vi "Simple Test.vi"() -> ()   [LabVIEW 2019, in "instrument.PPMS.lvclass"]
uses:
  instrument.PPMS.lvclass
  PPMS/Select PPMS--Enum.ctl
  PPMS/PPMS.lvlib
panel:
  out "x-y":dbl
  out "Temperature (K)":dbl
  in  "stop":bool
  in  "Select PPMS":T1=enum."Simulate PPMS"
  out "Paths":string
  out "getAll":variant
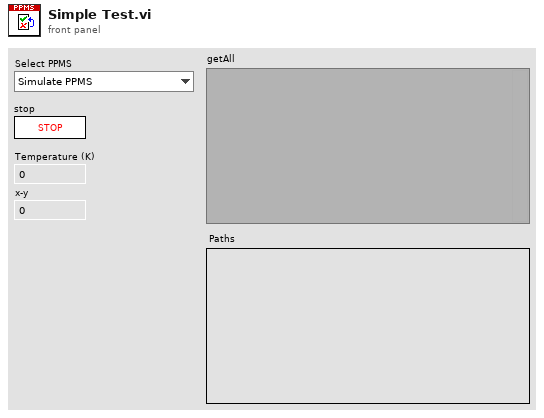
[diagram p1: front panel]
types:
  T1 = typedef "PPMS.lvlib/Select PPMS--Enum.ctl" = enum16{"PPMS1", "PPMS2", "PPMS3", "OptiCool", "Simulate PPMS", "Simulate OptiCool"}
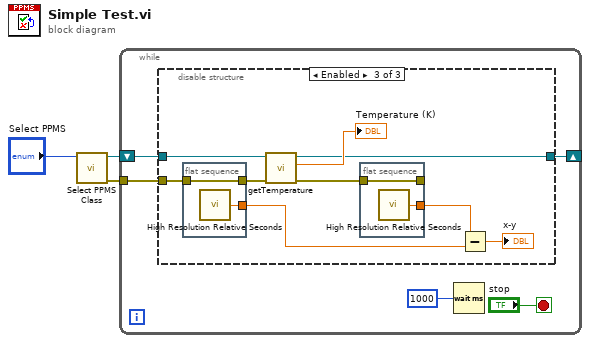
[diagram p0: block diagram]
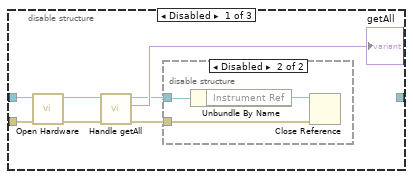
[diagram p2: hidden frame]
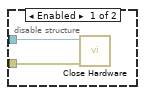
[diagram p3: hidden frame]
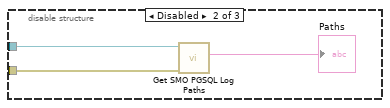
[diagram p4: hidden frame]
diagram:
  n1 = call "Select PPMS Class.vi"("Select PPMS"="Select PPMS") -> ("error out"=w2:errorcluster, "instrument.PPMS out"=w3:refnum<class "instrument.PPMS.lvclass">)  [unwired: 9 in]
  n2 = while {
    tunnel: w2 -> [w7]
    shift-right: [w5] -> _
    shift-left: w3 -> [w8]
    stop <- "stop" stop-if-true
    n3 = disable-structure shown="Enabled" {
      disable-tunnel: w8 -> [w15 w23 w32]
      disable-tunnel: w7 -> [w14 w22 w29]
      disable-tunnel: [_ _ w28] -> w5
      frame Disabled {
        n4 = call-dynamic "Open Hardware.vi"("error in (no error)"=w14, "instrument.PPMS"=w15) -> ("error out"=w12:errorcluster, "instrument.PPMS out"=w13:refnum<class "instrument.PPMS.lvclass">)  [unwired: 8 in]
        n5 = call-dynamic "Handle getAll.vi"("error in (no error)"=w12, "instrument.PPMS in"=w13) -> ("error out"=w11:errorcluster, "getAll"=→"getAll":variant, "instrument.PPMS out"=w9:refnum<class "instrument.PPMS.lvclass">)  [unwired: 7 in]
        n6 = disable-structure shown="Disabled" {
          disable-tunnel: w11 -> [w17 w20]
          disable-tunnel: w9 -> [w16 w19]
          frame Enabled {
            n7 = call-dynamic "Close Hardware.vi"("error in (no error)"=w17, "instrument.PPMS"=w16) -> ()  [unwired: 8 in, 2 out]
          }
          frame Disabled {
            n8 = Unbundle By Name(w19) -> ("Instrument Ref"=w18:refnum<k24>)
            n9 = Close Reference(reference=w18, error in (no error)=w20) -> ()  [unwired: 1 out]
          }
        }
      }
      frame Disabled {
        n10 = call-dynamic "Get SMO PGSQL Log Paths.vi"("error in (no error)"=w22, "Instrument in"=w23) -> ("Paths"=→"Paths":string)  [unwired: 7 in, 2 out]
      }
      frame Enabled {
        n11 = flat-sequence {
          tunnel: [w36] -> w30
          tunnel: w29 -> [w36]
          tunnel: [w35] -> w24
          frame #0 {
            n12 = call <vilib>:"High Resolution Relative Seconds.vi"() -> ("relative seconds"=w35:dbl)
          }
        }
        n13 = call-dynamic "getTemperature.vi"("error in (no error)"=w30, "instrument.PPMS"=w32) -> ("error out"=w27:errorcluster, "Temperature (K)"=→"Temperature (K)":dbl, "instrument.PPMS out"=w28:refnum<class "instrument.PPMS.lvclass">)  [unwired: 5 in, 2 out]
        n14 = flat-sequence {
          tunnel: [w34] -> _
          tunnel: w27 -> [w34]
          tunnel: [w33] -> w26
          frame #0 {
            n15 = call <vilib>:"High Resolution Relative Seconds.vi"() -> ("relative seconds"=w33:dbl)
          }
        }
        n16 = Subtract(x=w26, y=w24) -> (x-y=→"x-y":dbl)
      }
    }
    n17 = Wait (ms)(milliseconds to wait=u32 1000) -> ()  [unwired: 1 out]
  }
